vi "Destroy.vi"(11 "Dev Actor Panel in":refnum<class "Dev Panel.lvclass">) -> (0 "error out":errorcluster)   [LabVIEW 2021, in "Dev Panel.lvclass"]
uses:
  Dev Panel.lvclass
  Dev Panel.lvclass/Dev Panel.ctl
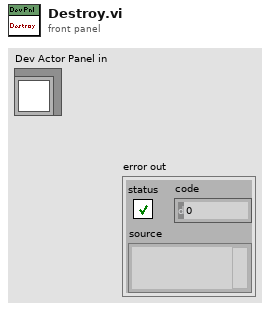
[diagram p1: front panel]
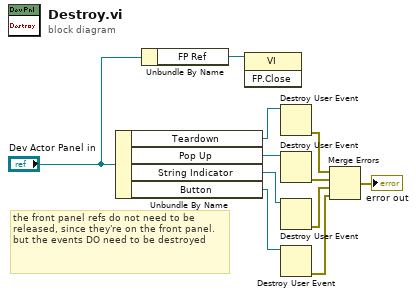
[diagram p0: block diagram]
diagram:
  # "the front panel refs do not need to be released, since they're on the front panel. but the events DO need to be destroyed"
  n1 = Unbundle By Name("Dev Actor Panel in") -> ("Teardown"=w11:refnum<user-event>, "Pop Up"=w9:refnum<user-event>, "String Indicator"=w6:refnum<user-event>, "Button"=w5:refnum<user-event>)
  n2 = Unbundle By Name("Dev Actor Panel in") -> ("FP Ref"=w1:refnum<vi>)
  n3 = invoke class="VI" method="FP.Close"(reference=w1) -> ()  [unwired: 2 in, 3 out]
  n4 = Destroy User Event(user event=w11) -> (error out=w10:errorcluster)  [unwired: 1 in]
  n5 = Destroy User Event(user event=w9) -> (error out=w7:errorcluster)  [unwired: 1 in]
  n6 = Destroy User Event(user event=w6) -> (error out=w4:errorcluster)  [unwired: 1 in]
  n7 = Destroy User Event(user event=w5) -> (error out=w3:errorcluster)  [unwired: 1 in]
  n8 = Merge Errors(w10, w7, w4, w3) -> (→"error out":errorcluster)
